vi "CAN Decode List File.vi"(8 "error in (no error)":errorcluster, 9 "IgnoreIDListLen":i32, 10 "pIgnoreIDList":u32, 11 "pFileName":string) -> (0 "error out":errorcluster, 1 "function return":i32, 2 "pIgnoreIDList out":u32, 3 "pFileName out":string)   [LabVIEW 2010, in "usb2an.lvlib"]
doc: "int WINAPI CAN_DecodeListFile(char *pFileName,unsigned int *pIgnoreIDList,int IgnoreIDListLen);"
uses:
  usb2an.lvlib
  USB2XXX.dll
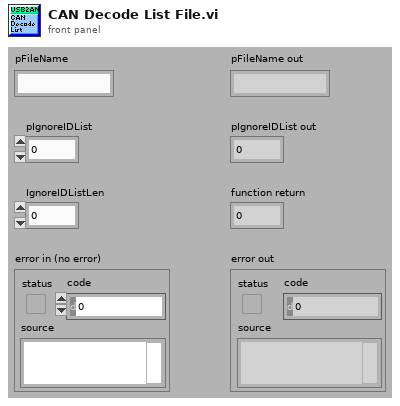
[diagram p1: front panel]
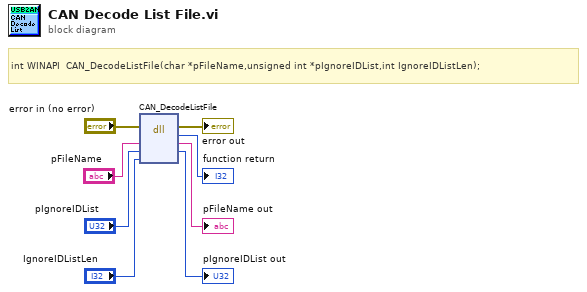
[diagram p0: block diagram]
diagram:
  # "int WINAPI  CAN_DecodeListFile(char *pFileName,unsigned int *pIgnoreIDList,int IgnoreIDListLen);"
  n1 = dll-call lib="E:/OtherWork/STM32/USB2XXX_Example/sdk/api/Labview/USB2XXX.*" fn="CAN_DecodeListFile"(error in="error in (no error)", "pFileName"="pFileName", "pIgnoreIDList"="pIgnoreIDList", "IgnoreIDListLen"="IgnoreIDListLen") -> (error out=→"error out":errorcluster, →"function return":i32, "pFileName"=→"pFileName out":string, "pIgnoreIDList"=→"pIgnoreIDList out":u32)  [unwired: 3 in, 1 out]
